vi "ConvertTimestamp.vi"(11 "Time Stamp":u32) -> (3 "Timestamp":timestamp)   [LabVIEW 2014]
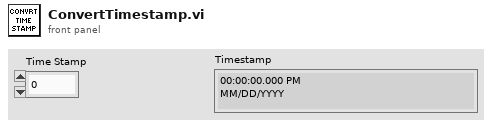
[diagram p1: front panel]
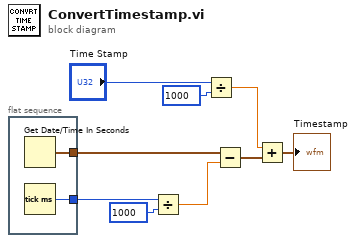
[diagram p0: block diagram]
diagram:
  n1 = flat-sequence {
    tunnel: [w11] -> w9
    tunnel: [w10] -> w5
    frame #0 {
      n2 = Get Date/Time In Seconds() -> (seconds since 1Jan1904=w11:timestamp)
      n3 = Tick Count (ms)() -> (millisecond timer value=w10:u32)
    }
  }
  n4 = Divide(x=w5, y=u64 1000) -> (x/y=w4:ext)
  n5 = Divide(x="Time Stamp", y=u64 1000) -> (x/y=w2:ext)
  n6 = Subtract(x=w9, y=w4) -> (x-y=w8:timestamp)
  n7 = Add(x=w2, y=w8) -> (x+y=→"Timestamp":timestamp)
